vi "Get Status.vi"(11 "Transfer Group in":refnum<class "Transfer Group.lvclass">) -> (2 "status pointer":refnum<class "Status Pointer.lvclass">, 3 "Transfer Group out":refnum<class "Transfer Group.lvclass">)   [LabVIEW 2019, in "DSF Core.lvlib" / "Transfer Group.lvclass"]
uses:
  Transfer Group.lvclass
  Status/Status Pointer.lvclass
  Transfer Group.lvclass/Transfer Group.ctl
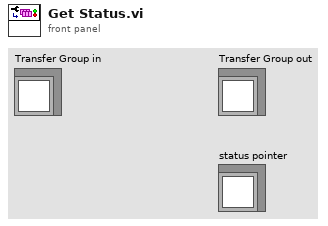
[diagram p1: front panel]
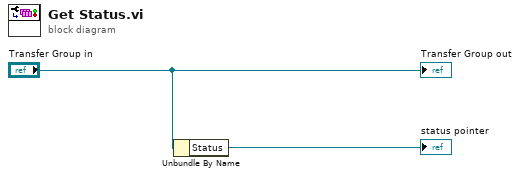
[diagram p0: block diagram]
diagram:
  n1 = Unbundle By Name("Transfer Group in") -> ("Status"=→"status pointer":refnum<class "Status Pointer.lvclass">)
  "Transfer Group out" <- "Transfer Group in"
